vi "Read Driver Joystick.vi"   [LabVIEW 2020]
uses:
  <vilib>/Rock Robotics/WPI/Utilities/WPI_GetSetVariantRefNum.vi
  <vilib>/Rock Robotics/Network Tables/NT Write Numeric Array.vi
  <vilib>/Rock Robotics/Network Tables/NT Write Boolean Array.vi
  Framework/Robot Global Data.vi
types:
  T1 = enum16{"0", "1", "2", "3", "4", "5", "6", "7", "8", "9", "10", "11"}
  T2 = typedef "WPI_JoystickDevRef.ctl" = cluster{"Device":T3}
  T3 = typedef "WPI_JoystickDeviceEnum.ctl" = enum16{"USB 0", "USB 1", "USB 2", "USB 3", "USB 4", "USB 5"}
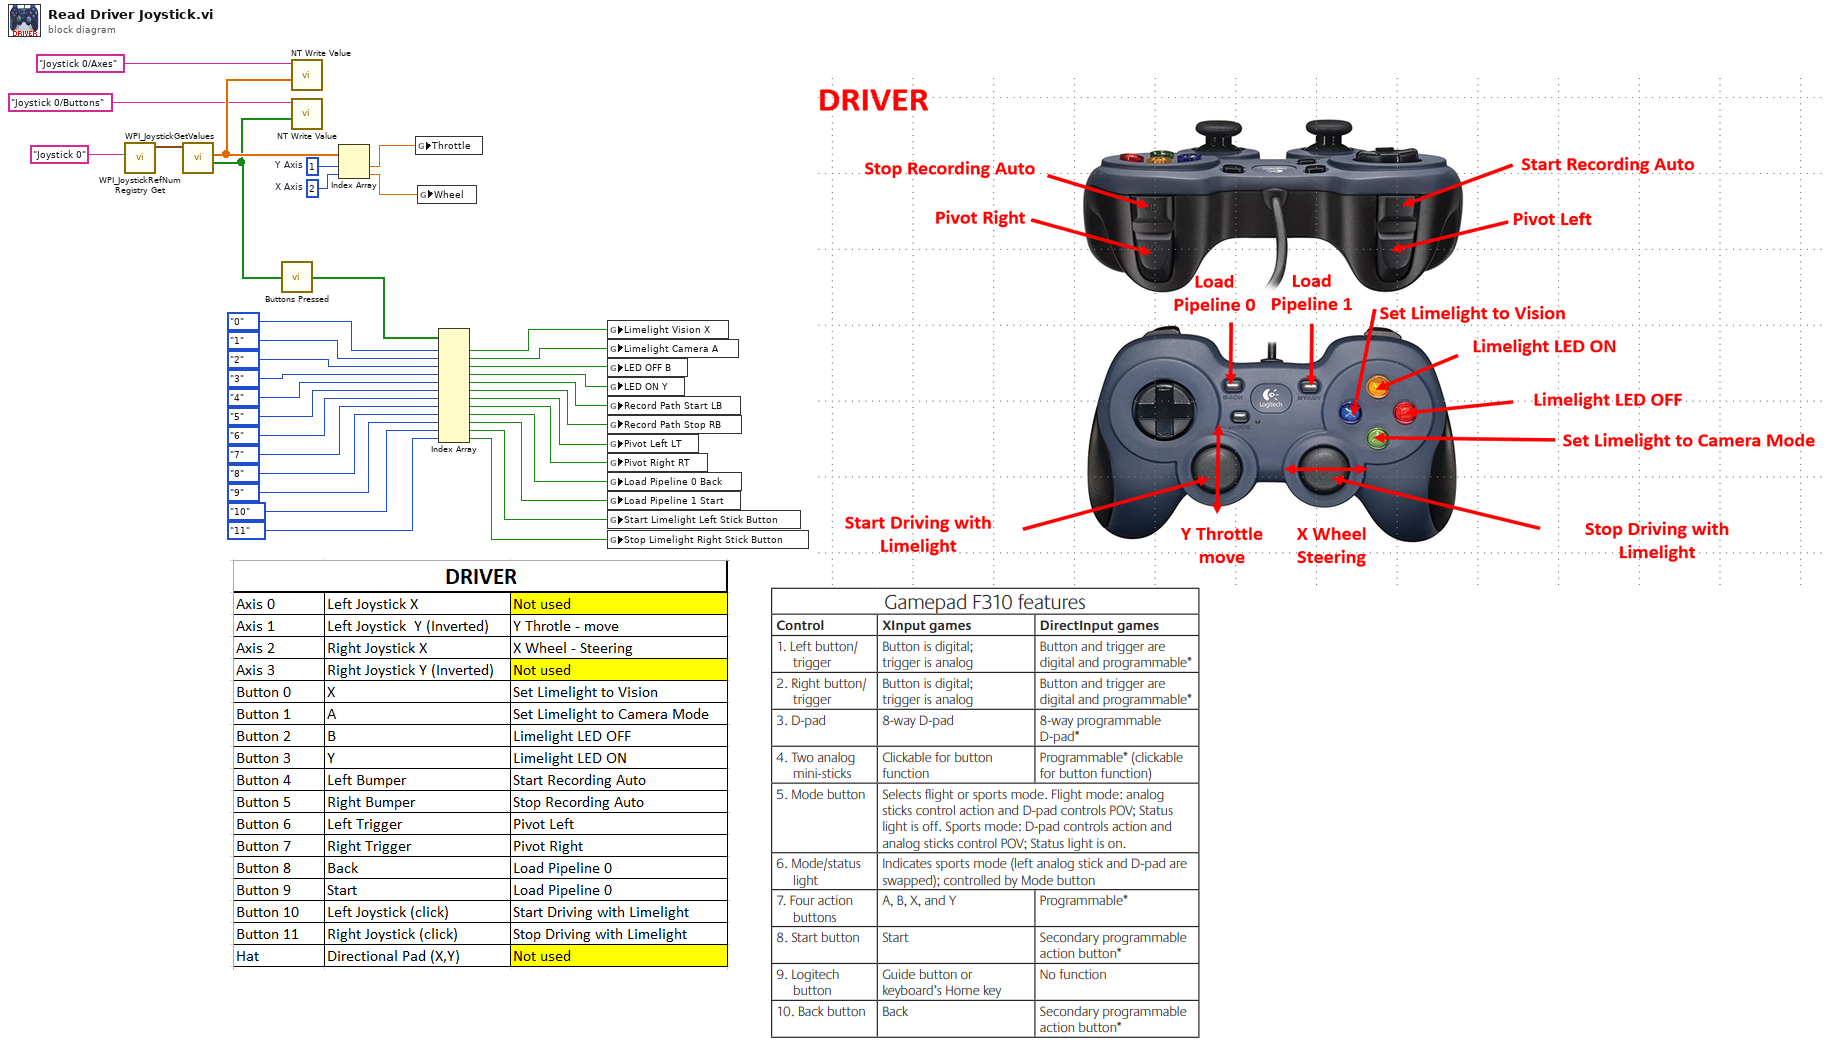
[diagram p0: block diagram]
diagram:
  w26 = 2  # X Axis
  w27 = 1  # Y Axis
  n1 = call <vilib>:"WPI_JoystickRefNum Registry Get.vi"("refnum name"="Joystick 0") -> ("JoystickDevRef"=w32:T2)  [unwired: 9 in, 1 out]
  n2 = call <vilib>:"WPI_JoystickGetValues.vi"("JoystickDevRef"=w32) -> ("Buttons"=w30:bool[], "Axes"=w35:dbl[])  [unwired: 6 in, 3 out]
  n3 = call "Buttons Pressed.vi"("Button Values"=w30) -> ("Button Presses"=w25:bool[])
  n4 = call-poly <vilib>:"NT Write Value.vi"("Numeric Array"=w35, "Name"="Joystick 0/Axes") -> ()  [unwired: 9 in, 1 out]
  n5 = call-poly <vilib>:"NT Write Value.vi"("Boolean Array"=w30, "Name"="Joystick 0/Buttons") -> ()  [unwired: 9 in, 1 out]
  n6 = Index Array(array=w35, index #1=w27, index #2=w26) -> (element #1=w29:dbl, element #2=w28:dbl)
  n7 = global write "Robot Global Data.vi" "Throttle"(w29) -> ()
  n8 = global write "Robot Global Data.vi" "Wheel"(w28) -> ()
  n9 = Index Array(array=w25, index #1=T1."0", index #2=T1."1", index #3=T1."2", index #4=T1."3", index #5=T1."4", index #6=T1."5", index #7=T1."6", index #8=T1."7", index #9=T1."8", index #10=T1."9", index #11=T1."10", index #12=T1."11") -> (element #1=w21:bool, element #2=w22:bool, element #3=w24:bool, element #4=w23:bool, element #5=w15:bool, element #6=w14:bool, element #7=w13:bool, element #8=w8:bool, element #9=w7:bool, element #10=w4:bool, element #11=w3:bool, element #12=w1:bool)
  n10 = global write "Robot Global Data.vi" "Limelight Vision X"(w21) -> ()
  n11 = global write "Robot Global Data.vi" "Limelight Camera A"(w22) -> ()
  n12 = global write "Robot Global Data.vi" "LED OFF B"(w24) -> ()
  n13 = global write "Robot Global Data.vi" "LED ON Y"(w23) -> ()
  n14 = global write "Robot Global Data.vi" "Record Path Start LB"(w15) -> ()
  n15 = global write "Robot Global Data.vi" "Record Path Stop RB"(w14) -> ()
  n16 = global write "Robot Global Data.vi" "Pivot Left LT"(w13) -> ()
  n17 = global write "Robot Global Data.vi" "Pivot Right RT"(w8) -> ()
  n18 = global write "Robot Global Data.vi" "Load Pipeline 0 Back"(w7) -> ()
  n19 = global write "Robot Global Data.vi" "Load Pipeline 1 Start"(w4) -> ()
  n20 = global write "Robot Global Data.vi" "Start Limelight Left Stick Button"(w3) -> ()
  n21 = global write "Robot Global Data.vi" "Stop Limelight Right Stick Button"(w1) -> ()
